vi "Parse Log File Name.vi"(11 "Log file name":string="LogFile_{Year}-{Month}-{Day}-{Hour}-{Minute}-{Second}.tdms") -> (3 "Parsed Log file name":string)   [LabVIEW 2021, in "XNET-CAN-Signal-Logger.lvlib"]
uses:
  XNET-CAN-Signal-Logger.lvlib
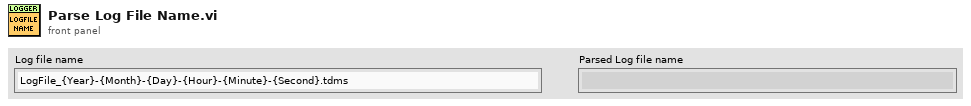
[diagram p1: front panel]
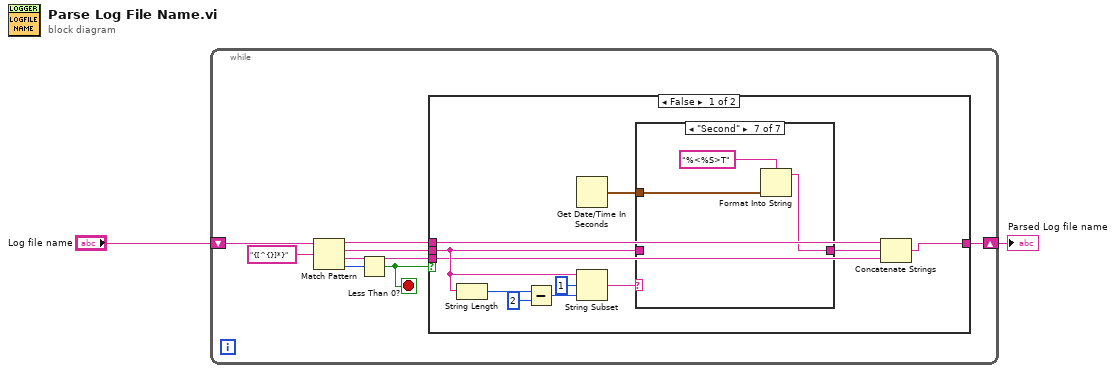
[diagram p0: block diagram]
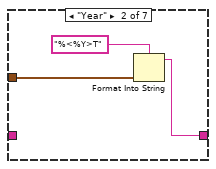
[diagram p3: hidden frame]
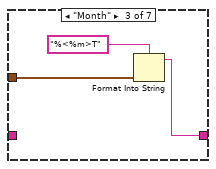
[diagram p4: hidden frame]
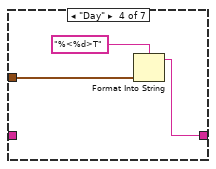
[diagram p5: hidden frame]
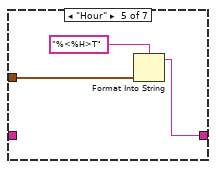
[diagram p6: hidden frame]
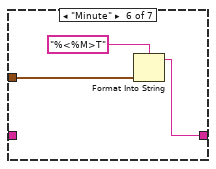
[diagram p7: hidden frame]
diagram:
  n1 = while {
    shift-right: [w3] -> w1
    shift-left: "Log file name" -> [w10]
    stop <- w6 stop-if-true
    n2 = Match Pattern(string=w10, regular expression="{[^{}]*}") -> (before substring=w5:string, match substring=w7:string, after substring=w4:string, offset past match=w8:i32)  [unwired: 1 in]
    n3 = Less Than 0?(x=w8) -> (x < 0?=w6:bool)
    n4 = case shown="False" w6 {
      tunnel: w7 -> [w15 _]
      tunnel: w5 -> [w14 w41]
      tunnel: w4 -> [w12 _]
      tunnel: [w11 w41] -> w3
      frame False {
        n5 = String Length(string=w15) -> (length=w20:i32)
        n6 = Subtract(x=w20, y=2) -> (x-y=w18:i32)
        n7 = Get Date/Time In Seconds() -> (seconds since 1Jan1904=w16:timestamp)
        n8 = String Subset(string=w15, offset (0)=1, length (rest)=w18) -> (substring=w21:string)
        n9 = case shown="\"Second\"" w21 {
          selector: w21 -> [w22 _ _ _ _ _ _]
          tunnel: w16 -> [_ w25 w28 w31 w34 w37 w40]
          tunnel: w15 -> [_ _ _ _ _ _ _]
          tunnel: [w22 w23 w26 w29 w32 w35 w38] -> w13
          frame Default {
          }
          frame "Year" {
            n10 = Format Into String(format string="%<%Y>T", w25) -> (resulting string=w23:string)  [unwired: 2 in, 1 out]
          }
          frame "Month" {
            n11 = Format Into String(format string="%<%m>T", w28) -> (resulting string=w26:string)  [unwired: 2 in, 1 out]
          }
          frame "Day" {
            n12 = Format Into String(format string="%<%d>T", w31) -> (resulting string=w29:string)  [unwired: 2 in, 1 out]
          }
          frame "Hour" {
            n13 = Format Into String(format string="%<%H>T", w34) -> (resulting string=w32:string)  [unwired: 2 in, 1 out]
          }
          frame "Minute" {
            n14 = Format Into String(format string="%<%M>T", w37) -> (resulting string=w35:string)  [unwired: 2 in, 1 out]
          }
          frame "Second" {
            n15 = Format Into String(format string="%<%S>T", w40) -> (resulting string=w38:string)  [unwired: 2 in, 1 out]
          }
        }
        n16 = Concatenate Strings(w14, w13, w12) -> (w11:string)
      }
      frame True {
      }
    }
  }
  "Parsed Log file name" <- w1
